vi "ImPro - Get Settings.vi"(7 "ImProSettings on File":T1, 8 "error in (no error)":errorcluster, 11 "output cluster":T2) -> (0 "error out":errorcluster, 3 "ImProSettings Relative":T1)   [LabVIEW 2023]
uses:
  Controls/ImPro - UI Refs.ctl
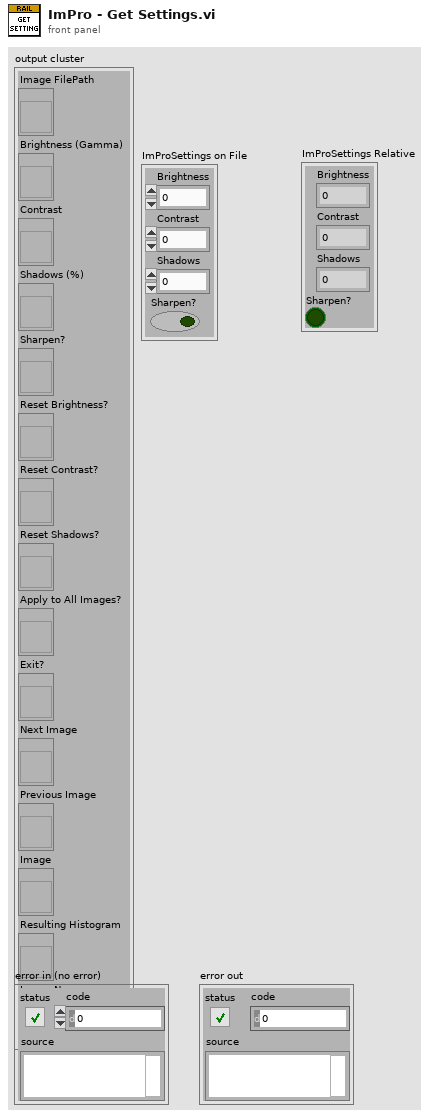
[diagram p1: front panel]
types:
  T1 = cluster{"Brightness":dbl, "Contrast":dbl, "Shadows":dbl, "Sharpen?":bool}
  T2 = typedef "ImPro - UI Refs.ctl" = cluster{"Image FilePath":refnum<vi>, "Brightness (Gamma)":refnum<vi>, "Contrast":refnum<vi>, "Shadows (%)":refnum<vi>, "Sharpen?":refnum<vi>, "Reset Brightness?":refnum<vi>, "Reset Contrast?":refnum<vi>, "Reset Shadows?":refnum<vi>, "Apply to All Images?":refnum<vi>, "Exit?":refnum<vi>, "Next Image":refnum<vi>, "Previous Image":refnum<vi>, "Image":refnum<vi>, "Resulting Histogram":refnum<vi>, "Image Name":refnum<vi>}
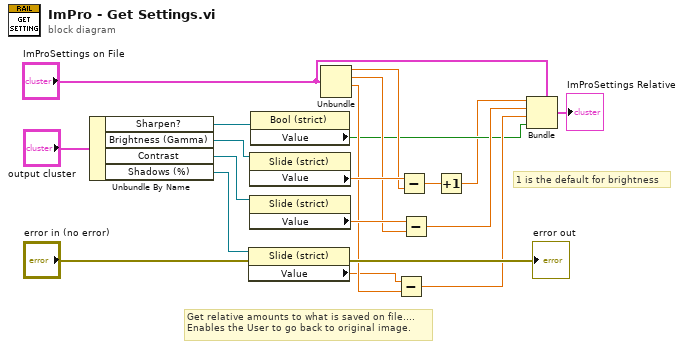
[diagram p0: block diagram]
diagram:
  # "1 is the default for brightness"
  # "Get relative amounts to what is saved on file....\nEnables the User to go back to original image."
  n1 = Unbundle By Name("output cluster") -> ("Sharpen?"=w20:refnum<vi>, "Brightness (Gamma)"=w19:refnum<vi>, "Contrast"=w18:refnum<vi>, "Shadows (%)"=w17:refnum<vi>)
  n2 = property class="Slide (strict)"(reference=w17, error in="error in (no error)") -> (error out=→"error out":errorcluster, "Value"=w10:dbl)  [unwired: 1 out]
  n3 = property class="Slide (strict)"(reference=w19) -> ("Value"=w13:dbl)  [unwired: 1 in, 2 out]
  n4 = property class="Slide (strict)"(reference=w18) -> ("Value"=w12:dbl)  [unwired: 1 in, 2 out]
  n5 = property class="Bool (strict)"(reference=w20) -> ("Value"=w3:bool)  [unwired: 1 in, 2 out]
  n6 = Unbundle("ImProSettings on File") -> ("Brightness"=w8:dbl, "Contrast"=w9:dbl, "Shadows"=w11:dbl)  [unwired: 1 out]
  n7 = Subtract(x=w10, y=w11) -> (x-y=w4:dbl)
  n8 = Subtract(x=w13, y=w8) -> (x-y=w6:dbl)
  n9 = Subtract(x=w12, y=w9) -> (x-y=w5:dbl)
  n10 = Increment(x=w6) -> (x+1=w1:dbl)
  n11 = Bundle(cluster="ImProSettings on File", "Brightness"=w1, "Contrast"=w5, "Shadows"=w4, "Sharpen?"=w3) -> (→"ImProSettings Relative":T1)
